vi "subvi_jenoptik_phase_fitting.vi"(0 "allow last extremum to be minimum?":bool, 2 "algorithm":enum16{"2nd order fit", "3rd order fit"}(ring), 7 "intensity":sgl[](array[numeric]) format="%.2f", 11 "error in (no error)":errorcluster) -> (8 "phase":dbl[](array[numeric]) format="%.2f", 15 "error out":errorcluster)   [LabVIEW 2019]
uses:
  <vilib>/Analysis/1siggen.llb/Ramp Pattern by Samples.vi
  <vilib>/Analysis/NI_AALPro.lvlib
  <vilib>/Analysis/NI_AALBase.lvlib
panel:
  out "Intensity":T1(graph)
  in  "extremum":T2={"type"=enum."maximum", "x"=0, "y"=0.0} {"y" format="%.2f"}
  # "--->"
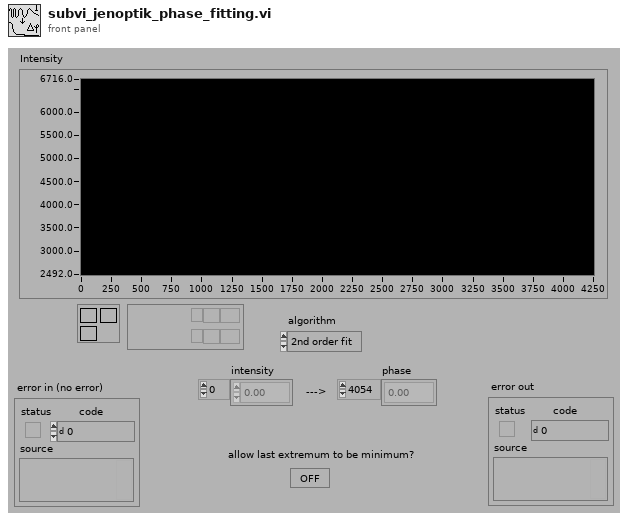
[diagram p1: front panel]
types:
  T1 = cluster{"Ramp Pattern":dbl[], "Best Polynomial Fit":dbl[]}[]
  T2 = cluster{"type":enum16{"minimum", "maximum"}, "x":i32, "y":dbl}
  T3 = cluster{"type":enum16{"minimum", "maximum"}, "x":i32, "y":dbl}[]
  T4 = cluster{"Extremum":enum16{"minimum", "maximum"}, i32, sgl}
  T5 = cluster{"Extremum":enum16{"minimum", "maximum"}, "x":i32, "y":dbl}[]
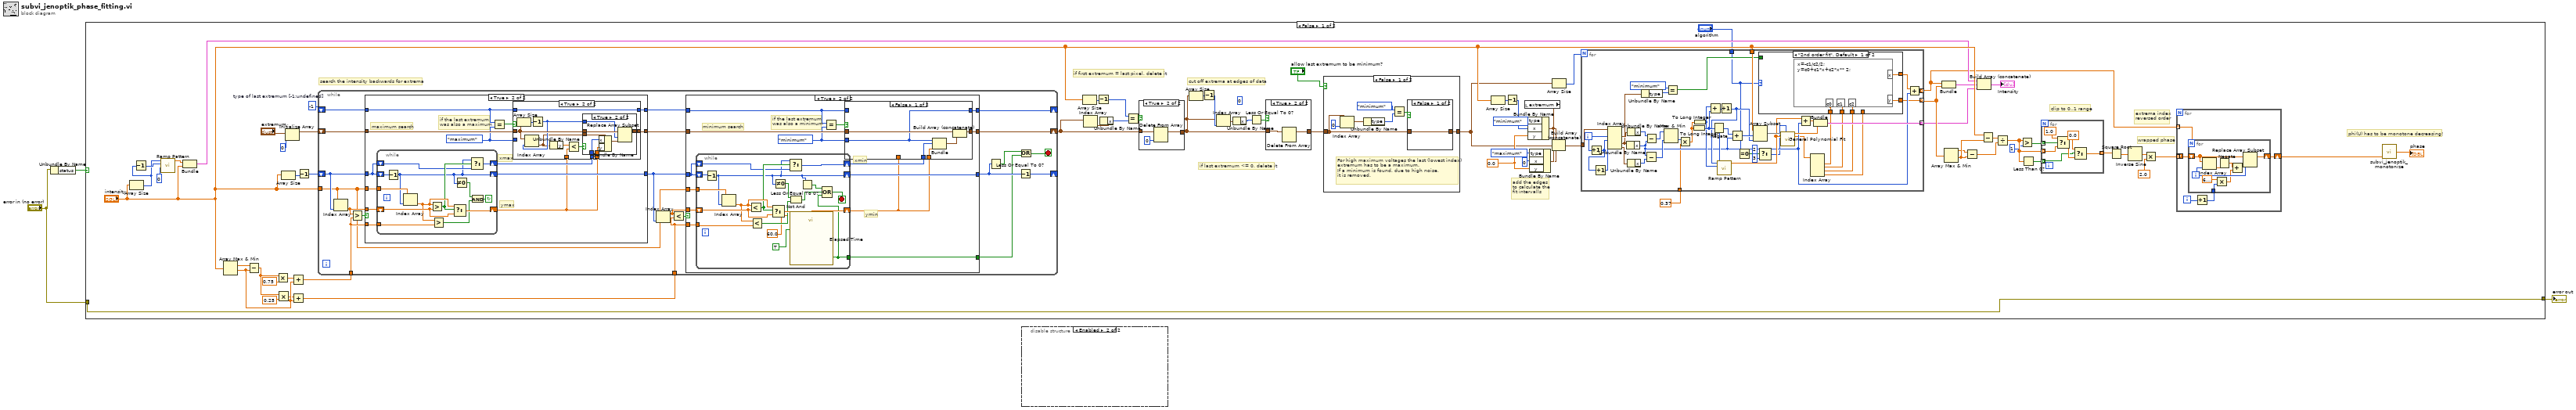
[diagram p0: block diagram]
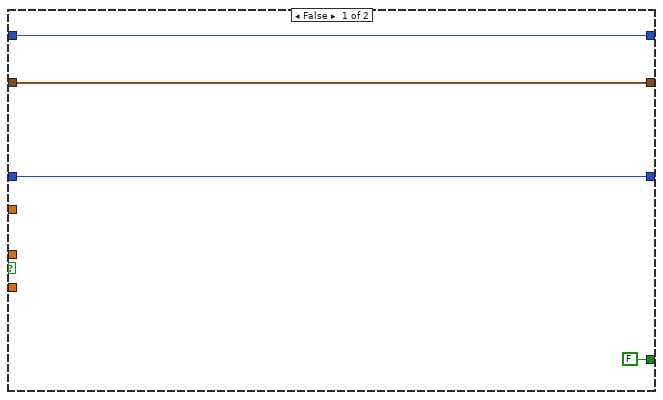
[diagram p3: hidden frame]
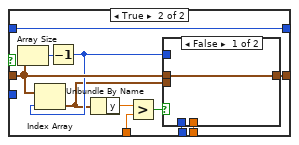
[diagram p4: hidden frame]
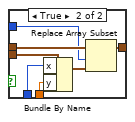
[diagram p5: hidden frame]
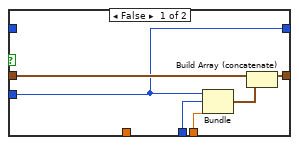
[diagram p7: hidden frame]
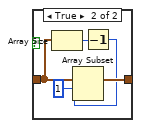
[diagram p9: hidden frame]
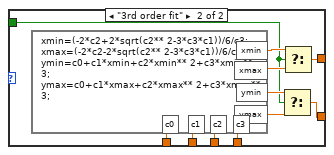
[diagram p11: hidden frame]
diagram:
  n1 = Unbundle By Name("error in (no error)") -> ("status"=w3:bool)
  n2 = case shown="False" w3 {
    tunnel: "error in (no error)" -> [w8 w310]
    tunnel: [w8 w310] -> w1
    frame False {
      (unwired) 0 ("y")
      w51 = -1  # type of last extremum [-1:undefined]
      w67 = 0.0
      # "if last extremum <= 0, delete it"
      # "if first extremum = last pixel, delete it"
      # "phi(U) has to be monotone decreasing!"
      # "cut off extrema at edges of data"
      # "clip to 0..1 range"
      # "extrema index\nreversed order"
      # "wrapped phase"
      # "search the intensity backwards for extrema"
      # "add the edges\nto calculate the\nfit intervalls"
      n3 = Array Size(array="intensity") -> (size(s)=w25:i32)
      n4 = Decrement(x=w25) -> (x-1=w26:i32)
      n5 = call-poly <vilib>:"Ramp Pattern.vi"("start"=i16 0, "end"=w26, "samples"=w25) -> ("Ramp Pattern"=w27:dbl[])  [unwired: 7 in, 1 out]
      n6 = Bundle("Ramp Pattern"=w27, "intensity"="intensity") -> (w34:cluster{"Ramp Pattern":dbl[], "intensity":sgl[]})  [unwired: 1 out]
      n7 = Array Max & Min(array="intensity") -> (max value=w12:sgl, min value=w53:sgl)  [unwired: 2 out]
      n8 = Subtract(x=w12, y=w53) -> (x-y=w52:sgl)
      n9 = Multiply(x=w52, y=sgl 0.75) -> (x*y=w13:sgl)
      n10 = Multiply(x=w52, y=sgl 0.25) -> (x*y=w15:sgl)
      n11 = Array Size(array="intensity") -> (size(s)=w17:i32)
      n12 = Initialize Array("extremum", 0 ("Dimension Size")) -> (w61:T3)
      n13 = Add(x=w13, y=w53) -> (x+y=w18:sgl)
      n14 = Add(x=w15, y=w53) -> (x+y=w19:sgl)
      n15 = Decrement(x=w17) -> (x-1=w22:i32)
      n16 = while {
        shift-left: w51 -> [w87]
        shift-right: [w82] -> _
        tunnel: w19 -> [w77]
        tunnel: w18 -> [w88]
        shift-left: w61 -> [w90]
        shift-right: [w81] -> w4
        tunnel: "intensity" -> [w80]
        shift-left: w22 -> [w92]
        shift-right: [w89] -> _
        stop <- w74 stop-if-true
        n17 = Index Array(array=w80, index=w92) -> (element=w91:sgl)
        n18 = Greater?(x=w91, y=w88) -> (0:w93:bool)
        n19 = case shown="True" w93 {
          tunnel: w80 -> [_ w170]
          tunnel: w92 -> [w157 w167]
          tunnel: [w157 w168] -> w84
          tunnel: w88 -> [_ w169]
          tunnel: w91 -> [_ w166]
          tunnel: w90 -> [w156 w164]
          tunnel: [w156 w163] -> w85
          tunnel: w87 -> [w155 w161]
          tunnel: [w155 w162] -> w86
          frame False {
          }
          frame True {
            w160 = enum16{"minimum", "maximum"}."maximum" ("Extremum")
            # "if the last extremum\nwas also a maximum"
            # "xmax"
            # "ymax"
            # "maximum search"
            n20 = while {
              shift-left: w167 -> [w172]
              shift-right: [w173] -> w165
              shift-left: w166 -> [w180]
              shift-right: [w179] -> w158
              tunnel: w169 -> [w181]
              shift-left: w167 -> [w183]
              shift-right: [w171] -> w168
              tunnel: w170 -> [w182]
              stop <- w176 continue-if-true
              n21 = Decrement(x=w183) -> (x-1=w171:i32)
              n22 = Index Array(array=w182, index=w171) -> (element=w175:sgl)
              n23 = Greater?(x=w175, y=w180) -> (0:w174:bool)
              n24 = Greater?(x=w175, y=w181) -> (0:w177:bool)
              n25 = Select(t=w175, s=w174, f=w180) -> (s? t:f=w179:sgl)
              n26 = Not Equal To 0?(x=w171) -> (x != 0?=w178:bool)
              n27 = Select(t=w171, s=w174, f=w172) -> (s? t:f=w173:i32)
              n28 = And(x=w178, y=w177) -> (x .and. y?=w176:bool)
            }
            n29 = Equal?(x=w161, y=w160) -> (x = y?=w159:bool)
            n30 = case shown="True" w159 {
              tunnel: w165 -> [w187 w192]
              tunnel: w164 -> [w189 w197]
              tunnel: [w188 w195] -> w163
              tunnel: w158 -> [w186 w198]
              tunnel: w161 -> [_ w190]
              tunnel: [w184 w190] -> w162
              tunnel: w160 -> [w184 _]
              tunnel: w158 -> [_ w194]
              frame False {
                n31 = Bundle("Extremum"=w184, w187, w186) -> (w185:T4)  [unwired: 1 out]
                n32 = Build Array (concatenate)(w189, w185) -> (w188:T5)
              }
              frame True {
                n33 = Array Size(array=w197) -> (size(s)=w200:i32)
                n34 = Decrement(x=w200) -> (x-1=w193:i32)
                n35 = Index Array(array=w197, index=w193) -> (element=w191:T2)
                n36 = Unbundle By Name(w191) -> ("y"=w199:dbl)
                n37 = Less?(x=w199, y=w194) -> (x < y?=w196:bool)
                n38 = case shown="True" w196 {
                  tunnel: w197 -> [w201 w208]
                  tunnel: [w201 w207] -> w195
                  tunnel: w193 -> [_ w206]
                  tunnel: w192 -> [_ w203]
                  tunnel: w198 -> [_ w202]
                  tunnel: w191 -> [_ w205]
                  frame False {
                  }
                  frame True {
                    n39 = Bundle By Name(cluster=w205, "x"=w203, "y"=w202) -> (w204:T2)
                    n40 = Replace Array Subset(array=w208, new element=w204, index=w206) -> (w207:T3)
                  }
                }
              }
            }
          }
        }
        n41 = Index Array(array=w80, index=w84) -> (element=w79:sgl)
        n42 = Less?(x=w79, y=w77) -> (x < y?=w78:bool)
        n43 = case shown="True" w78 {
          tunnel: w80 -> [_ w111]
          tunnel: w84 -> [w97 w108]
          tunnel: [w97 w109] -> w83
          tunnel: w77 -> [_ w110]
          tunnel: w79 -> [_ w107]
          tunnel: w85 -> [w96 w105]
          tunnel: [w96 w104] -> w81
          tunnel: w86 -> [w95 w102]
          tunnel: [w95 w103] -> w82
          tunnel: [FALSE ("Time has Elapsed") w98] -> w75
          frame False {
          }
          frame True {
            w101 = enum16{"minimum", "maximum"}."minimum" ("Extremum")
            # "if the last extremum\nwas also a minimum"
            # "xmin"
            # "ymin"
            # "minimum search"
            n44 = while {
              shift-left: w108 -> [w119]
              shift-right: [w120] -> w106
              shift-left: w107 -> [w126]
              shift-right: [w125] -> w99
              tunnel: w110 -> [w127]
              shift-left: w108 -> [w129]
              shift-right: [w113] -> w109
              tunnel: w111 -> [w128]
              tunnel: [w114] -> w98
              stop <- w115 stop-if-true
              n45 = Decrement(x=w129) -> (x-1=w113:i32)
              n46 = Index Array(array=w128, index=w113) -> (element=w122:sgl)
              n47 = Less?(x=w122, y=w126) -> (x < y?=w121:bool)
              n48 = Less?(x=w122, y=w127) -> (x < y?=w123:bool)
              n49 = Select(t=w122, s=w121, f=w126) -> (s? t:f=w125:sgl)
              n50 = Not Equal To 0?(x=w113) -> (x != 0?=w124:bool)
              n51 = Select(t=w113, s=w121, f=w119) -> (s? t:f=w120:i32)
              n52 = Not And(1:w123, 2:w124) -> (0:w116:bool)
              n53 = call "Elapsed Time"("Time Target (s)"=60.0, "Auto Reset"=TRUE) -> ("Time has Elapsed"=w114:bool)  [unwired: 10 in, 7 out]
              n54 = Less Or Equal To 0?(x=w113) -> (x <= 0?=w112:bool)
              n55 = Compound Arithmetic op=OR(w112, w116, w114) -> (w115:bool)
            }
            n56 = Equal?(x=w102, y=w101) -> (x = y?=w100:bool)
            n57 = case shown="False" w100 {
              tunnel: w106 -> [w133 w138]
              tunnel: w105 -> [w135 w143]
              tunnel: [w134 w141] -> w104
              tunnel: w99 -> [w132 w144]
              tunnel: w102 -> [_ w136]
              tunnel: [w130 w136] -> w103
              tunnel: w101 -> [w130 _]
              tunnel: w99 -> [_ w140]
              frame False {
                n58 = Bundle("Extremum"=w130, w133, w132) -> (w131:T4)  [unwired: 1 out]
                n59 = Build Array (concatenate)(w135, w131) -> (w134:T5)
              }
              frame True {
                n60 = Array Size(array=w143) -> (size(s)=w146:i32)
                n61 = Decrement(x=w146) -> (x-1=w139:i32)
                n62 = Index Array(array=w143, index=w139) -> (element=w137:T2)
                n63 = Unbundle By Name(w137) -> ("y"=w145:dbl)
                n64 = Greater?(x=w145, y=w140) -> (0:w142:bool)
                n65 = case shown="False" w142 {
                  tunnel: w143 -> [w147 w154]
                  tunnel: [w147 w153] -> w141
                  tunnel: w139 -> [_ w152]
                  tunnel: w138 -> [_ w149]
                  tunnel: w144 -> [_ w148]
                  tunnel: w137 -> [_ w151]
                  frame False {
                  }
                  frame True {
                    n66 = Bundle By Name(cluster=w151, "x"=w149, "y"=w148) -> (w150:T2)
                    n67 = Replace Array Subset(array=w154, new element=w150, index=w152) -> (w153:T3)
                  }
                }
              }
            }
          }
        }
        n68 = Less Or Equal To 0?(x=w83) -> (x <= 0?=w76:bool)
        n69 = Decrement(x=w83) -> (x-1=w89:i32)
        n70 = Or(x=w76, y=w75) -> (x .or. y?=w74:bool)
      }
      n71 = Array Size(array="intensity") -> (size(s)=w20:i32)
      n72 = Index Array(array=w4) -> (element=w47:T2)  [unwired: 1 in]
      n73 = Decrement(x=w20) -> (x-1=w23:i32)
      n74 = Unbundle By Name(w47) -> ("x"=w48:i32)
      n75 = Equal?(x=w23, y=w48) -> (x = y?=w55:bool)
      n76 = case shown="True" w55 {
        tunnel: [w303 w305] -> w56
        tunnel: w4 -> [w303 w306]
        frame False {
        }
        frame True {
          n77 = Delete From Array(array=w306, index=0) -> (array with subset deleted=w305:T3)  [unwired: 1 in, 1 out]
        }
      }
      n78 = Array Size(array=w56) -> (size(s)=w21:i32)
      n79 = Decrement(x=w21) -> (x-1=w59:i32)
      n80 = Index Array(array=w56, index=w59) -> (element=w49:T2)
      n81 = Unbundle By Name(w49) -> ("x"=w50:i32)
      n82 = Less Or Equal To 0?(x=w50) -> (x <= 0?=w58:bool)
      n83 = case shown="True" w58 {
        tunnel: [w307 w308] -> w57
        tunnel: w56 -> [w307 w309]
        frame False {
        }
        frame True {
          n84 = Delete From Array(array=w309) -> (array with subset deleted=w308:T3)  [unwired: 2 in, 1 out]
        }
      }
      n85 = case shown="False" "allow last extremum to be minimum?" {
        tunnel: [w215 w222] -> w60
        tunnel: w57 -> [w214 w222]
        frame False {
          # "For high maximum voltages the last (lowest index)\nextremum has to be a maximum.\nIf a minimum is found, due to high noise,\nit is removed."
          n86 = Index Array(array=w214, index=0 ("Index")) -> (element=w209:T2)
          n87 = Unbundle By Name(w209) -> ("type"=w211:enum16{"minimum", "maximum"})
          n88 = Equal?(x=enum16{"minimum", "maximum"}."minimum" ("Output Element"), y=w211) -> (x = y?=w213:bool)
          n89 = case shown="False" w213 {
            tunnel: w214 -> [w216 w217]
            tunnel: [w216 w220] -> w215
            frame False {
            }
            frame True {
              n90 = Array Size(array=w217) -> (size(s)=w219:i32)
              n91 = Decrement(x=w219) -> (x-1=w218:i32)
              n92 = Array Subset(array=w217, index=1 ("Array Index"), length=w218) -> (w220:T3)
            }
          }
        }
        frame True {
          # "for low voltages the first extremum\ncan be an maximum"
        }
      }
      n93 = Array Size(array="intensity") -> (size(s)=w30:i32)
      n94 = Decrement(x=w30) -> (x-1=w69:i32)
      n95 = local read "extremum"() -> (w65:T2)
      n96 = Bundle By Name(cluster=w65, "type"=enum16{"minimum", "maximum"}."minimum" ("Bundle Element"), "x"=w69, "y"=w67) -> (w66:T2)
      n97 = Bundle By Name(cluster=w65, "type"=enum16{"minimum", "maximum"}."maximum" ("Bundle Element"), "x"=0 ("Input Element"), "y"=w67) -> (w64:T2)
      n98 = Build Array (concatenate)(w66, w60, w64) -> (w31:T3)
      n99 = Array Size(array=w60) -> (size(s)=w32:i32)
      n100 = for {
        N: w32 -> [_]
        tunnel: "intensity" -> [w265]
        tunnel: [w261] -> w28 mode=indexing
        tunnel: w31 -> [w258]
        tunnel: 0.37 -> [w238]
        tunnel: [w242] -> w54 mode=indexing
        tunnel: [w252] -> w10 mode=indexing
        tunnel: "algorithm" -> [w232]
        i -> [w259]
        n101 = Increment(x=w259) -> (x+1=w231:i32)
        n102 = Increment(x=w231) -> (x+1=w230:i32)
        n103 = Index Array(array=w258, index #1=w259, index #2=w231, index #4=w230) -> (element #1=w251:T2, element #3=w228:T2, element #4=w229:T2)  [unwired: 1 in, 1 out]
        n104 = Unbundle By Name(w228) -> ("x"=w244:i32)
        n105 = Unbundle By Name(w251) -> ("x"=w250:i32)
        n106 = Unbundle By Name(w229) -> ("x"=w249:i32)
        n107 = Unbundle By Name(w228) -> ("type"=w240:enum16{"minimum", "maximum"})
        n108 = Subtract(x=w244, y=w249) -> (x-y=w257:i32)
        n109 = Subtract(x=w250, y=w244) -> (x-y=w237:i32)
        n110 = Max & Min(x=w237, y=w257) -> (min(x,y)=w254:i32)  [unwired: 1 out]
        n111 = Equal?(x=enum16{"minimum", "maximum"}."minimum" ("Output Element"), y=w240) -> (x = y?=w239:bool)
        n112 = Multiply(x=w254, y=w238) -> (x*y=w236:dbl)
        n113 = To Long Integer(number=w236) -> (32bit integer=w256:i32)
        n114 = To Long Integer(number=w236) -> (32bit integer=w248:i32)
        n115 = Add(x=w248, y=w256) -> (x+y=w255:i32)
        n116 = Negate(x=w256) -> (-x=w247:i32)
        n117 = Increment(x=w255) -> (x+1=w245:i32)
        n118 = call-poly <vilib>:"Ramp Pattern.vi"("start"=w247, "end"=w248, "samples"=w245) -> ("Ramp Pattern"=w260:dbl[])  [unwired: 7 in, 1 out]
        n119 = Add(x=w247, y=w244) -> (x+y=w246:i32)
        n120 = Equal To 0?(x=w232) -> (x = 0?=w233:bool)
        n121 = Array Subset(array=w265, index=w246, length=w245) -> (w264:sgl[])
        n122 = Select(t=i16 2, s=w233, f=i16 3) -> (s? t:f=w223:i16)
        n123 = call <vilib>:"General Polynomial Fit.vi"("Y"=w264, "polynomial order"=w223, "X"=w260) -> ("Best Polynomial Fit"=w262:dbl[], "Polynomial Coefficients"=w224:dbl[])  [unwired: 9 in, 2 out]
        n124 = Add(x=w260, y=w244) -> (x+y=w263:dbl[])
        n125 = Index Array(array=w224) -> (element #1=w253:dbl, element #2=w227:dbl, element #3=w226:dbl, element #4=w225:dbl)  [unwired: 4 in]
        n126 = case shown="\"2nd order fit\", Default" w232 {
          tunnel: w253 -> [w269 w281]
          tunnel: w227 -> [w270 w280]
          tunnel: w225 -> [_ w279]
          tunnel: [w268 w276] -> w243
          tunnel: [w267 w273] -> w242
          tunnel: w239 -> [_ w272]
          tunnel: w226 -> [w266 w271]
          frame "2nd order fit", Default {
            n127 = formula code="x=-c1/c2/2;\ny=c0+c1*x+c2*x** 2;"("c0"=w269, "c2"=w266, "c1"=w270) -> ("x"=w268:dbl, "y"=w267:dbl)
          }
          frame "3rd order fit" {
            n128 = formula code="xmin=(-2*c2+2*sqrt(c2** 2-3*c3*c1))/6/c3;\nxmax=(-2*c2-2*sqrt(c2** 2-3*c3*c1))/6/c3;\nymin=c0+c1*xmin+c2*xmin** 2+c3*xmin** 3;\nymax=c0+c1*xmax+c2*xmax** 2+c3*xmax** 3;"("c0"=w281, "c1"=w280, "c2"=w271, "c3"=w279) -> ("ymax"=w274:dbl, "xmax"=w277:dbl, "xmin"=w278:dbl, "ymin"=w275:dbl)
            n129 = Select(t=w275, s=w272, f=w274) -> (s? t:f=w273:dbl)
            n130 = Select(t=w278, s=w272, f=w277) -> (s? t:f=w276:dbl)
          }
        }
        n131 = Bundle(w263, "Best Polynomial Fit"=w262) -> (w261:cluster{dbl[], "Best Polynomial Fit":dbl[]})  [unwired: 1 out]
        n132 = Add(x=w243, y=w244) -> (x+y=w252:dbl)
      }
      n133 = Bundle(w10, w54) -> (w72:cluster{dbl[], dbl[]})  [unwired: 1 out]
      n134 = Array Max & Min(array=w54) -> (max value=w35:dbl, min value=w36:dbl)  [unwired: 2 out]
      n135 = Subtract(x=w35, y=w36) -> (x-y=w38:dbl)
      n136 = Build Array (concatenate)(w34, w72, w28) -> (→"Intensity":T1)
      n137 = Subtract(x="intensity", y=w36) -> (x-y=w37:dbl[])
      n138 = Divide(x=w37, y=w38) -> (x/y=w41:dbl[])
      n139 = Greater?(x=w41, y=1) -> (0:w40:bool[])
      n140 = Less Than 0?(x=w41) -> (x < 0?=w42:bool[])
      n141 = for {
        tunnel: w40 -> [w288] mode=indexing
        tunnel: w41 -> [w286] mode=indexing
        tunnel: w42 -> [w284] mode=indexing
        tunnel: [w282] -> w43 mode=indexing
        n142 = Select(t=1.0, s=w288, f=w286) -> (s? t:f=w285:dbl)
        n143 = Select(t=0.0, s=w284, f=w285) -> (s? t:f=w282:dbl)
      }
      n144 = Square Root(x=w43) -> (sqrt(x)=w44:dbl[])
      n145 = Inverse Sine(1:w44) -> (0:w45:dbl[])
      n146 = Multiply(x=w45, y=2.0 ("t")) -> (x*y=w6:dbl[])
      n147 = for {
        shift-right: [w293] -> w5
        shift-left: w6 -> [w292]
        tunnel: [w292] -> _ mode=indexing
        tunnel: w10 -> [w289] mode=indexing
        i -> [w291]
        n148 = Increment(x=w291) -> (x+1=w290:i32)
        n149 = for {
          N: w289 -> [_]
          shift-right: [w300] -> w293
          shift-left: w292 -> [w301]
          tunnel: w290 -> [w295]
          i -> [w302]
          n150 = Index Array(array=w301, index=w302) -> (element=w299:dbl)
          n151 = Multiply(x=6.283185307179586, y=w295) -> (x*y=w294:dbl)
          n152 = Negate(x=w299) -> (-x=w298:dbl)
          n153 = Add(x=w298, y=w294) -> (x+y=w297:dbl)
          n154 = Replace Array Subset(array=w301, new element=w297, index=w302) -> (w300:dbl[])
        }
      }
      n155 = call "subvi_jenoptik_monotonize.vi"("Array"=w5) -> ("phase"=→"phase":dbl[])
    }
    frame True {
    }
  }
  "error out" <- w1
  n156 = disable-structure shown="Enabled" {
    frame Disabled {
    }
    frame Enabled {
    }
  }
